vi "listen for analogue loop commands.vi"(7 "RT Queues":T2, 11 "Analogue loop data":T1) -> (1 "Analogue FIFO states out":T3, 3 "Analogue loop data":T1)   [LabVIEW 2018]
uses:
  Analogue FIFO loop states.ctl
  Chris VIs/Incident logger/Incidents/Warning/Warning.lvclass
  Queue VIs/De-queue RT message element.vi
  Z:/OneDrive - Imperial College London/LabVIEW/Chris VIs/Incident logger/Incidents/Incident.lvclass
  Type Defs/Queues cluster.ctl
  Type Defs/Analogue loop data.ctl
  Chris VIs/Message Scheduler/message scheduler.lvclass
panel:
  out "Message received":string
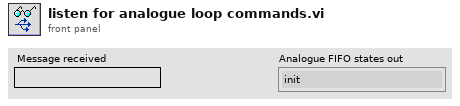
[diagram p1: front panel]
types:
  T1 = typedef "Analogue loop data.ctl" = cluster{"Params":cluster{"FPGA Ref":refnum<k20>, "Channels":u32, "FIFO Depth":u32}, "Variables":cluster{"Last read":u32}}
  T2 = typedef "Queues cluster.ctl" = cluster{"RT Message":refnum<queue>, "RT Comms":refnum<queue>, "RT Data":refnum<queue>, "message scheduler":refnum<class "message scheduler.lvclass">}
  T3 = typedef "Analogue FIFO loop states.ctl" = enum16{"init", "connect", "read", "stop", "quit"}
  T4 = cluster{"Target":string, "Loop":string, "Code":string}
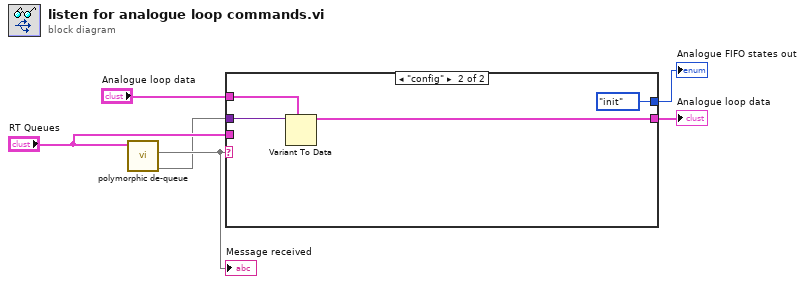
[diagram p0: block diagram]
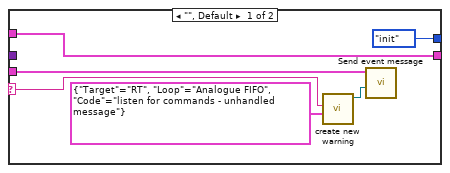
[diagram p2: hidden frame]
diagram:
  n1 = call-poly "polymorphic de-queue.vi"("RT Queues"="RT Queues") -> (0:w3, 2:w4)  [unwired: 7 in, 2 out]
  "Message received" <- w4
  n2 = case shown="\"config\"" w4 {
    selector: w4 -> [w8 _]
    tunnel: "RT Queues" -> [w12 _]
    tunnel: [Analogue_FIFO_loop_states."init" ("Analogue FIFO states in") Analogue_FIFO_loop_states."init" ("Analogue FIFO states in")] -> w6
    tunnel: w3 -> [_ w15]
    tunnel: "Analogue loop data" -> [w11 w14]
    tunnel: [w11 w13] -> w1
    frame "", Default {
      n3 = call "create new warning.vi"("Location"=T4 {"Target"="RT", "Loop"="Analogue FIFO", "Code"="listen for commands - unhandled message"}, "Description"=w8) -> ("Warning out"=w9:refnum<class "Warning.lvclass">)  [unwired: 8 in, 1 out]
      n4 = call "Send event message.vi"("Incident"=w9, "RT Queues"=w12) -> ()  [unwired: 10 in]
    }
    frame "config" {
      n5 = Variant To Data(type=w14, Variant=w15) -> (data=w13:T1)  [unwired: 1 in, 1 out]
    }
  }
  "Analogue FIFO states out" <- w6
  "Analogue loop data" <- w1
